vi "RGseriesSeria170309org.vi"() -> ()   [LabVIEW 2015]
uses:
  <vilib>/Instr/_visa.llb/VISA Configure Serial Port (Instr).vi
  <userlib>/caLab/Private/Get_PV.vi
panel:
  out "PS2:R_MV":dbl format="%.2f"
  out "PS1:R_MV":dbl format="%.2f"
  out "number 2":dbl
  out "number":dbl
  out "APX:Tpiezo":dbl
  in  "REMOTE/LOCAL":bool
  out "APX:Thpc":dbl
  in  "Reset Timer2":bool=TRUE caption="Auto Reset"
  in  "Time Target2 (min)":dbl=1.0 caption="Time Target (s)"
  out "Elapsed Time2 (min)":dbl caption="Elapsed Time (s)"
  out "Time has Elapsed 2":bool caption="Time has Elapsed"
  in  "Timer2":bool
  in  "Timer1":bool
  in  "Reset Timer1":bool=TRUE caption="Auto Reset"
  out "Time has Elapsed":bool
  in  "Time Target1 (min)":dbl=1.0 caption="Time Target (s)"
  out "Elapsed Time (min)":dbl caption="Elapsed Time (s)"
  in  "PS1:I_RV":dbl min=0.0 max=0.5 step=0.01
  in  "PS1:V_RV":dbl min=0.0 max=5.0 step=0.01
  out "PS1:P_MV":dbl format="%.2f"
  out "PS1:I_MV":dbl format="%.3g"
  out "PS1:V_MV":dbl format="%.3g"
  in  "PS1:OUT":bool
  out "APX:Thpc OK?":bool
  out "APX:Tpiezo OK?":bool
  out "PS2:P_MV":dbl format="%.2f"
  in  "PS2:I_RV":dbl min=0.0 max=2.3 step=0.02
  in  "PS2:OUT":bool
  in  "stop":bool
  out "PS2:I_MV":dbl format="%.3g"
  out "APX:PS2_V_MV":dbl format="%.3g"
  in  "VISA resource name":refnum<visa-resource-name>="COM12"
  in  "PS2:V_RV":dbl min=0.0 max=3.3 step=0.05
  # "COM12"
  # "Sample Heater Control"
  # "HPC Heater Control"
  # "V"
  # "V"
  # "A"
  # "A"
  # "Max 1.2A/0.4x0.1wire"
  # "W"
  # "ohm"
  # "W"
  # "ohm"
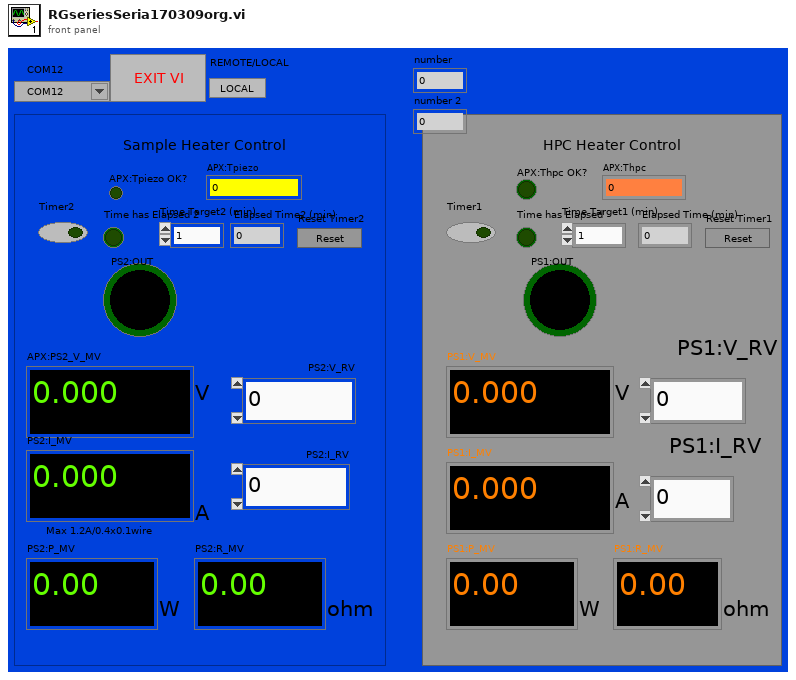
[diagram p1: front panel]
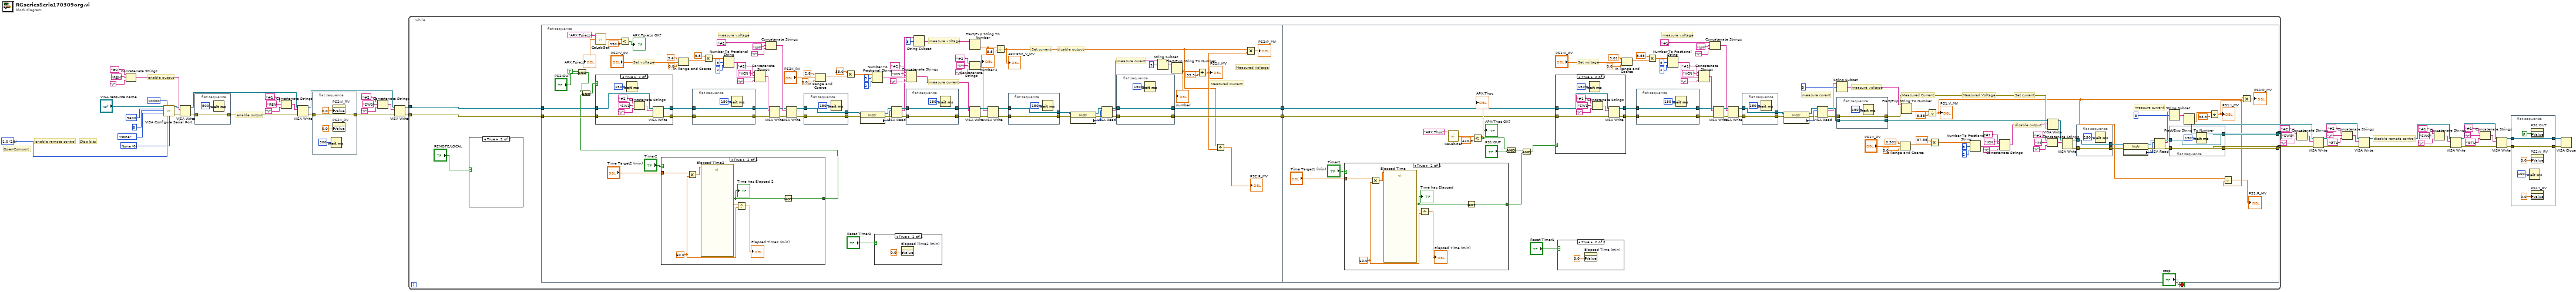
[diagram p0: block diagram]
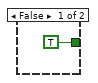
[diagram p4: hidden frame]
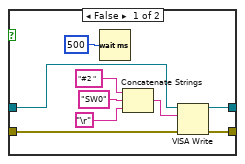
[diagram p5: hidden frame]
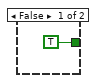
[diagram p7: hidden frame]
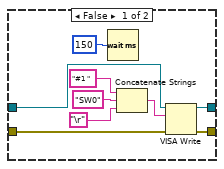
[diagram p8: hidden frame]
diagram:
  w44 = u16 0 items=["None", "XON/XOFF", "RTS/CTS", "XON/XOFF & RTS/CTS", "DTR/DSR", "XON/XOFF & DTR/DSR"] ("flow control (0:none)")
  w45 = u16 10 items=["1.0"=10, "1.5"=15, "2.0"=20] ("stop bits (10: 1 bit)")
  # "enable output"
  # "disable remote control"
  # "OpenComport"
  # "Stop bits"
  # "enable remote control"
  # "enable output"
  n1 = Concatenate Strings("#2 " ("initial string"), "REN" ("string"), "\r") -> (w43:string)
  n2 = call-poly "VISA Configure Serial Port"("VISA resource name"="VISA resource name", "timeout (10sec)"=u32 10000, "baud rate (9600)"=u32 9600, "data bits (8)"=u16 8, "parity (0:none)"=enum16{"None", "Odd", "Even", "Mark", "Space"}."None", "stop bits (10: 1 bit)"=w45, "flow control (0:none)"=w44) -> ("VISA resource name out"=w40:refnum<visa-resource-name>, "error out"=w39:errorcluster)  [unwired: 7 in]
  n3 = VISA Write(VISA resource name=w40, write buffer=w43, error in (no error)=w39) -> (VISA resource name out=w9:refnum<visa-resource-name>, error out=w2:errorcluster)  [unwired: 1 out]
  n4 = flat-sequence {
    tunnel: w2 -> [w59]
    tunnel: [w59] -> w3
    frame #0 {
      n5 = Wait (ms)(milliseconds to wait=u32 500) -> ()  [unwired: 1 out]
    }
  }
  n6 = Concatenate Strings("#1 " ("initial string"), "REN" ("string"), "\r") -> (w4:string)
  n7 = VISA Write(VISA resource name=w9, write buffer=w4, error in (no error)=w3) -> (VISA resource name out=w8:refnum<visa-resource-name>, error out=w1:errorcluster)  [unwired: 1 out]
  n8 = flat-sequence {
    tunnel: [w63] -> w26
    tunnel: w1 -> [w63]
    frame #0 {
      n9 = Wait (ms)(milliseconds to wait=u32 500) -> ()  [unwired: 1 out]
      n10 = property on="PS2:V_RV" class="DigNum (strict)"("Value"=0.0 ("VCN_REQ")) -> ()  [unwired: 2 in, 2 out]
      n11 = property on="PS2:I_RV" class="DigNum (strict)"("Value"=0.0 ("APX:RG183_I_RV")) -> ()  [unwired: 2 in, 2 out]
    }
  }
  n12 = Concatenate Strings("#2 " ("format string"), "SW0" ("initial string"), "\r" ("input 1")) -> (w42:string)
  n13 = VISA Write(VISA resource name=w8, write buffer=w42, error in (no error)=w26) -> (VISA resource name out=w28:refnum<visa-resource-name>, error out=w27:errorcluster)  [unwired: 1 out]
  n14 = while {
    tunnel: w28 -> [w70]
    tunnel: w27 -> [w71]
    tunnel: [w67] -> w25
    tunnel: [w66] -> w24
    stop <- "stop" stop-if-true
    n15 = case shown="True" "REMOTE/LOCAL" {
      frame False {
      }
      frame True {
      }
    }
    n16 = flat-sequence {
      tunnel: w71 -> [w99]
      tunnel: w70 -> [w97]
      tunnel: [w101] -> w69
      tunnel: [w100] -> w68
      tunnel: w69 -> [w243]
      tunnel: w68 -> [w240]
      tunnel: [w220] -> w67
      tunnel: [w219] -> w66
      frame #0 {
        # "measure current"
        # "measure voltage"
        # "measure voltage"
        # "measure curent"
        # "Measured Voltage"
        # "Measured Current"
        # "Set current"
        # "Set voltage"
        # "disable output"
        n17 = And(x=TRUE, y="PS2:OUT") -> (x .and. y?=w79:bool)
        n18 = call-poly <userlib>:"CaLabGet.vi"("PV Name"="APX:Tpiezo") -> ("1rst Value (number)"=w85:dbl)  [unwired: 8 in, 6 out]
        "APX:Tpiezo" <- w85
        n19 = Less?(x=w85, y=350.0) -> (x < y?=→"APX:Tpiezo OK?":bool)
        n20 = case shown="True" "Timer2" {
          tunnel: "Time Target2 (min)" -> [_ w167]
          tunnel: [TRUE w166] -> w77
          frame False {
          }
          frame True {
            w171 = 60.0 ("y")
            n21 = Multiply(x=w167, y=w171) -> (x*y=w169:dbl)
            n22 = call "Elapsed Time2"("Time Target (s)"=w169) -> ("Elapsed Time (s)"=w170:dbl, "Time has Elapsed"=w168:bool)  [unwired: 11 in, 6 out]
            "Time has Elapsed 2" <- w168
            n23 = Divide(x=w170, y=w171) -> (x/y=→"Elapsed Time2 (min)":dbl)
            n24 = Not(x=w168) -> (.not. x?=w166:bool)
          }
        }
        n25 = And(x=w79, y=w77) -> (x .and. y?=w76:bool)
        n26 = case shown="True" w76 {
          tunnel: w97 -> [w176 w185]
          tunnel: w99 -> [w175 w184]
          tunnel: [w174 w183] -> w98
          tunnel: [w173 w182] -> w96
          frame False {
            n27 = Wait (ms)(milliseconds to wait=u32 500) -> ()  [unwired: 1 out]
            n28 = Concatenate Strings("#2 " ("format string"), "SW0" ("initial string"), "\r" ("input 1")) -> (w178:string)
            n29 = VISA Write(VISA resource name=w176, write buffer=w178, error in (no error)=w175) -> (VISA resource name out=w173:refnum<visa-resource-name>, error out=w174:errorcluster)  [unwired: 1 out]
          }
          frame True {
            n30 = Wait (ms)(milliseconds to wait=u32 150) -> ()  [unwired: 1 out]
            n31 = Concatenate Strings("#2 " ("format string"), "SW1" ("initial string"), "\r" ("input 1")) -> (w187:string)
            n32 = VISA Write(VISA resource name=w185, write buffer=w187, error in (no error)=w184) -> (VISA resource name out=w182:refnum<visa-resource-name>, error out=w183:errorcluster)  [unwired: 1 out]
          }
        }
        n33 = In Range and Coerce(upper limit=3.6, x="PS2:V_RV", lower limit=0.0) -> (coerced(x)=w92:dbl)  [unwired: 1 out]
        n34 = flat-sequence {
          tunnel: w96 -> [w203]
          tunnel: w98 -> [w204]
          tunnel: [w204] -> w102
          tunnel: [w203] -> w103
          frame #0 {
            n35 = Wait (ms)(milliseconds to wait=u32 150) -> ()  [unwired: 1 out]
          }
        }
        n36 = Multiply(x=5.5, y=w92) -> (x*y=w161:dbl)
        n37 = Number To Fractional String(number=w161, width (-)=i16 5, precision (6)=i16 2) -> (F-format string=w162:string)  [unwired: 1 in]
        n38 = Concatenate Strings("#2" ("format string"), "VCN " ("initial string"), w162, "\r") -> (w107:string)
        n39 = Concatenate Strings("#2 " ("format string"), "VM" ("initial string"), "\r" ("input 1")) -> (w138:string)
        n40 = VISA Write(VISA resource name=w103, write buffer=w107, error in (no error)=w102) -> (VISA resource name out=w137:refnum<visa-resource-name>, error out=w136:errorcluster)  [unwired: 1 out]
        n41 = VISA Write(VISA resource name=w137, write buffer=w138, error in (no error)=w136) -> (VISA resource name out=w123:refnum<visa-resource-name>, error out=w121:errorcluster)  [unwired: 1 out]
        n42 = flat-sequence {
          tunnel: w123 -> [w202]
          tunnel: [w202] -> w122
          tunnel: w121 -> [w201]
          tunnel: [w201] -> w120
          frame #0 {
            n43 = Wait (ms)(milliseconds to wait=u32 150) -> ()  [unwired: 1 out]
          }
        }
        n44 = In Range and Coerce(upper limit=2.8, x="PS2:I_RV", lower limit=0.0) -> (coerced(x)=w88:dbl)  [unwired: 1 out]
        n45 = Multiply(x=33.0, y=w88) -> (x*y=w151:dbl)
        n46 = property class="Instr"(reference=w122, error in=w120) -> (reference out=w129:refnum<visa-resource-name>, error out=w128:errorcluster, "Serial Settings:Number of Bytes at Serial Port"=w127:u32)
        n47 = Number To Fractional String(number=w151, width (-)=i16 5, precision (6)=i16 2) -> (F-format string=w154:string)  [unwired: 1 in]
        n48 = case shown="True" "Reset Timer2" {
          frame False {
          }
          frame True {
            n49 = property on="Elapsed Time2 (min)" class="DigNum (strict)"("Value"=0.0 ("Elapsed Time (min)")) -> ()  [unwired: 2 in, 2 out]
          }
        }
        n50 = VISA Read(VISA resource name=w129, byte count=w127, error in (no error)=w128) -> (VISA resource name out=w115:refnum<visa-resource-name>, read buffer=w108:string, error out=w114:errorcluster)  [unwired: 1 out]
        n51 = flat-sequence {
          tunnel: w115 -> [w195]
          tunnel: w114 -> [w194]
          tunnel: [w195] -> w112
          tunnel: [w194] -> w113
          frame #0 {
            n52 = Wait (ms)(milliseconds to wait=u32 150) -> ()  [unwired: 1 out]
          }
        }
        n53 = Concatenate Strings("#2 " ("initial string"), "ICN " ("initial string"), w154, "\r") -> (w106:string)
        n54 = String Subset(string=w108, offset (0)=3) -> (substring=w105:string)  [unwired: 1 in]
        n55 = Concatenate Strings("#2 " ("format string"), "IM" ("initial string"), "\r" ("input 1")) -> (w131:string)
        n56 = Fract/Exp String To Number(string=w105) -> (number=w147:dbl)  [unwired: 3 in, 1 out]
        "number 2" <- w147
        n57 = VISA Write(VISA resource name=w112, write buffer=w106, error in (no error)=w113) -> (VISA resource name out=w133:refnum<visa-resource-name>, error out=w134:errorcluster)  [unwired: 1 out]
        n58 = VISA Write(VISA resource name=w133, write buffer=w131, error in (no error)=w134) -> (VISA resource name out=w119:refnum<visa-resource-name>, error out=w118:errorcluster)  [unwired: 1 out]
        n59 = Divide(x=w147, y=5.5 ("x")) -> (x/y=w74:dbl)
        "APX:PS2_V_MV" <- w74
        n60 = flat-sequence {
          tunnel: w119 -> [w198]
          tunnel: w118 -> [w197]
          tunnel: [w198] -> w117
          tunnel: [w197] -> w116
          frame #0 {
            n61 = Wait (ms)(milliseconds to wait=u32 150) -> ()  [unwired: 1 out]
          }
        }
        n62 = property class="Instr"(reference=w117, error in=w116) -> (reference out=w126:refnum<visa-resource-name>, error out=w125:errorcluster, "Serial Settings:Number of Bytes at Serial Port"=w124:u32)
        n63 = VISA Read(VISA resource name=w126, byte count=w124, error in (no error)=w125) -> (VISA resource name out=w111:refnum<visa-resource-name>, read buffer=w109:string, error out=w110:errorcluster)  [unwired: 1 out]
        n64 = flat-sequence {
          tunnel: w111 -> [w192]
          tunnel: w110 -> [w191]
          tunnel: [w192] -> w101
          tunnel: [w191] -> w100
          frame #0 {
            n65 = Wait (ms)(milliseconds to wait=u32 150) -> ()  [unwired: 1 out]
          }
        }
        n66 = String Subset(string=w109, offset (0)=3) -> (substring=w104:string)  [unwired: 1 in]
        n67 = Fract/Exp String To Number(string=w104) -> (number=w144:dbl)  [unwired: 3 in, 1 out]
        "number" <- w144
        n68 = Divide(x=w144, y=33.5 ("x")) -> (x/y=w75:dbl)
        "PS2:I_MV" <- w75
        n69 = Divide(x=w74, y=w75) -> (x/y=→"PS2:R_MV":dbl)
        n70 = Multiply(x=w74, y=w75) -> (x*y=→"PS2:P_MV":dbl)
      }
      frame #1 {
        # "measure curent"
        # "Measured Voltage"
        # "Measured Current"
        # "disable output"
        # "measure current"
        # "measure voltage"
        # "Set current"
        # "measure voltage"
        # "Set voltage"
        n71 = case shown="True" "Timer1" {
          tunnel: "Time Target1 (min)" -> [_ w299]
          tunnel: [TRUE w298] -> w210
          frame False {
          }
          frame True {
            w303 = 60.0 ("y")
            n72 = Multiply(x=w299, y=w303) -> (x*y=w301:dbl)
            n73 = call "Elapsed Time"("Time Target (s)"=w301) -> ("Elapsed Time (s)"=w302:dbl, "Time has Elapsed"=w300:bool)  [unwired: 11 in, 6 out]
            "Time has Elapsed" <- w300
            n74 = Divide(x=w302, y=w303) -> (x/y=→"Elapsed Time (min)":dbl)
            n75 = Not(x=w300) -> (.not. x?=w298:bool)
          }
        }
        n76 = call-poly <userlib>:"CaLabGet.vi"("PV Name"="APX:Thpc") -> ("1rst Value (number)"=w294:dbl)  [unwired: 8 in, 6 out]
        "APX:Thpc" <- w294
        n77 = Less?(x=w294, y=420.0) -> (x < y?=w242:bool)
        "APX:Thpc OK?" <- w242
        n78 = And(x=w242, y="PS1:OUT") -> (x .and. y?=w214:bool)
        n79 = And(x=w214, y=w210) -> (x .and. y?=w213:bool)
        n80 = case shown="True" w213 {
          tunnel: w243 -> [w317 w326]
          tunnel: w240 -> [w316 w325]
          tunnel: [w315 w324] -> w239
          tunnel: [w314 w323] -> w238
          frame False {
            n81 = Wait (ms)(milliseconds to wait=u32 150) -> ()  [unwired: 1 out]
            n82 = Concatenate Strings("#1 " ("format string"), "SW0" ("initial string"), "\r" ("input 1")) -> (w321:string)
            n83 = VISA Write(VISA resource name=w317, write buffer=w321, error in (no error)=w316) -> (VISA resource name out=w314:refnum<visa-resource-name>, error out=w315:errorcluster)  [unwired: 1 out]
          }
          frame True {
            n84 = Wait (ms)(milliseconds to wait=u32 150) -> ()  [unwired: 1 out]
            n85 = Concatenate Strings("#1 " ("format string"), "SW1" ("initial string"), "\r" ("input 1")) -> (w330:string)
            n86 = VISA Write(VISA resource name=w326, write buffer=w330, error in (no error)=w325) -> (VISA resource name out=w323:refnum<visa-resource-name>, error out=w324:errorcluster)  [unwired: 1 out]
          }
        }
        n87 = case shown="True" "Reset Timer1" {
          frame False {
          }
          frame True {
            n88 = property on="Elapsed Time (min)" class="DigNum (strict)"("Value"=0.0 ("Elapsed Time (min)")) -> ()  [unwired: 2 in, 2 out]
          }
        }
        n89 = In Range and Coerce(upper limit=5.01, x="PS1:V_RV", lower limit=0.0) -> (coerced(x)=w255:dbl)  [unwired: 1 out]
        n90 = flat-sequence {
          tunnel: [w333] -> w236
          tunnel: w239 -> [w333]
          tunnel: [w332] -> w237
          tunnel: w238 -> [w332]
          frame #0 {
            n91 = Wait (ms)(milliseconds to wait=u32 150) -> ()  [unwired: 1 out]
          }
        }
        n92 = Multiply(x=5.55, y=w255) -> (x*y=w246:dbl)
        n93 = Number To Fractional String(number=w246, width (-)=i16 5, precision (6)=i16 2) -> (F-format string=w245:string)  [unwired: 1 in]
        n94 = Concatenate Strings("#1" ("format string"), "VCN " ("initial string"), w245, "\r") -> (w260:string)
        n95 = Concatenate Strings("#1" ("format string"), "VM" ("initial string"), "\r" ("input 1")) -> (w259:string)
        n96 = VISA Write(VISA resource name=w237, write buffer=w260, error in (no error)=w236) -> (VISA resource name out=w261:refnum<visa-resource-name>, error out=w288:errorcluster)  [unwired: 1 out]
        n97 = VISA Write(VISA resource name=w261, write buffer=w259, error in (no error)=w288) -> (VISA resource name out=w289:refnum<visa-resource-name>, error out=w290:errorcluster)  [unwired: 1 out]
        n98 = flat-sequence {
          tunnel: w289 -> [w337]
          tunnel: [w337] -> w291
          tunnel: w290 -> [w336]
          tunnel: [w336] -> w292
          frame #0 {
            n99 = Wait (ms)(milliseconds to wait=u32 150) -> ()  [unwired: 1 out]
          }
        }
        n100 = property class="Instr"(reference=w291, error in=w292) -> (reference out=w284:refnum<visa-resource-name>, error out=w285:errorcluster, "Serial Settings:Number of Bytes at Serial Port"=w286:u32)
        n101 = VISA Read(VISA resource name=w284, byte count=w286, error in (no error)=w285) -> (VISA resource name out=w218:refnum<visa-resource-name>, read buffer=w287:string, error out=w216:errorcluster)  [unwired: 1 out]
        n102 = String Subset(string=w287, offset (0)=3) -> (substring=w276:string)  [unwired: 1 in]
        n103 = flat-sequence {
          tunnel: w218 -> [w307]
          tunnel: [w307] -> w217
          tunnel: [w305] -> w215
          tunnel: w216 -> [w305]
          frame #0 {
            n104 = Wait (ms)(milliseconds to wait=u32 150) -> ()  [unwired: 1 out]
          }
        }
        n105 = In Range and Coerce(upper limit=0.501, x="PS1:I_RV", lower limit=0.0) -> (coerced(x)=w280:dbl)  [unwired: 1 out]
        n106 = Fract/Exp String To Number(string=w276) -> (number=w270:dbl)  [unwired: 3 in, 1 out]
        n107 = Divide(x=w270, y=5.55 ("x")) -> (x/y=w208:dbl)
        "PS1:V_MV" <- w208
        n108 = Multiply(x=37.35, y=w280) -> (x*y=w266:dbl)
        n109 = Number To Fractional String(number=w266, width (-)=i16 5, precision (6)=i16 2) -> (F-format string=w263:string)  [unwired: 1 in]
        n110 = Concatenate Strings("#1 " ("initial string"), "ICN " ("initial string"), w263, "\r") -> (w281:string)
        n111 = Concatenate Strings("#1 " ("format string"), "IM" ("initial string"), "\r" ("input 1")) -> (w282:string)
        n112 = VISA Write(VISA resource name=w217, write buffer=w281, error in (no error)=w215) -> (VISA resource name out=w283:refnum<visa-resource-name>)  [unwired: 2 out]
        n113 = VISA Write(VISA resource name=w283, write buffer=w282) -> (VISA resource name out=w223:refnum<visa-resource-name>, error out=w222:errorcluster)  [unwired: 1 in, 1 out]
        n114 = flat-sequence {
          tunnel: w223 -> [w312]
          tunnel: w222 -> [w311]
          tunnel: [w312] -> w229
          tunnel: [w311] -> w228
          frame #0 {
            n115 = Wait (ms)(milliseconds to wait=u32 150) -> ()  [unwired: 1 out]
          }
        }
        n116 = property class="Instr"(reference=w229, error in=w228) -> (reference out=w232:refnum<visa-resource-name>, error out=w231:errorcluster, "Serial Settings:Number of Bytes at Serial Port"=w230:u32)
        n117 = VISA Read(VISA resource name=w232, byte count=w230, error in (no error)=w231) -> (VISA resource name out=w227:refnum<visa-resource-name>, read buffer=w225:string, error out=w226:errorcluster)  [unwired: 1 out]
        n118 = String Subset(string=w225, offset (0)=3) -> (substring=w224:string)  [unwired: 1 in]
        n119 = flat-sequence {
          tunnel: w227 -> [w309]
          tunnel: w226 -> [w308]
          tunnel: [w309] -> w220
          tunnel: [w308] -> w219
          frame #0 {
            n120 = Wait (ms)(milliseconds to wait=u32 150) -> ()  [unwired: 1 out]
          }
        }
        n121 = Fract/Exp String To Number(string=w224) -> (number=w234:dbl)  [unwired: 3 in, 1 out]
        n122 = Divide(x=w234, y=33.3 ("x")) -> (x/y=w207:dbl)
        "PS1:I_MV" <- w207
        n123 = Divide(x=w208, y=w207) -> (x/y=→"PS1:R_MV":dbl)
        n124 = Multiply(x=w208, y=w207) -> (x*y=→"PS1:P_MV":dbl)
      }
    }
  }
  n125 = Concatenate Strings("#2 " ("format string"), "SW0" ("initial string"), "\r" ("input 1")) -> (w34:string)
  n126 = VISA Write(VISA resource name=w25, write buffer=w34, error in (no error)=w24) -> (VISA resource name out=w30:refnum<visa-resource-name>, error out=w29:errorcluster)  [unwired: 1 out]
  n127 = Concatenate Strings("#2 " ("initial string"), "\r", "GTL" ("input 1")) -> (w41:string)
  n128 = VISA Write(VISA resource name=w30, write buffer=w41, error in (no error)=w29) -> (VISA resource name out=w13:refnum<visa-resource-name>, error out=w12:errorcluster)  [unwired: 1 out]
  n129 = Concatenate Strings("#1 " ("format string"), "SW0" ("initial string"), "\r" ("input 1")) -> (w19:string)
  n130 = VISA Write(VISA resource name=w13, write buffer=w19, error in (no error)=w12) -> (VISA resource name out=w15:refnum<visa-resource-name>, error out=w14:errorcluster)  [unwired: 1 out]
  n131 = Concatenate Strings("#1" ("initial string"), "\r", "GTL" ("input 1")) -> (w20:string)
  n132 = VISA Write(VISA resource name=w15, write buffer=w20, error in (no error)=w14) -> (VISA resource name out=w11:refnum<visa-resource-name>, error out=w10:errorcluster)  [unwired: 1 out]
  n133 = flat-sequence {
    tunnel: w11 -> [w342]
    tunnel: w10 -> [w341]
    tunnel: [w342] -> w36
    tunnel: [w341] -> w35
    frame #0 {
      n134 = Wait (ms)(milliseconds to wait=u32 100) -> ()  [unwired: 1 out]
      n135 = property on="PS2:OUT" class="Bool (strict)"("Value"=FALSE ("Output")) -> ()  [unwired: 2 in, 2 out]
      n136 = property on="PS2:V_RV" class="DigNum (strict)"("Value"=0.0 ("VCN_REQ")) -> ()  [unwired: 2 in, 2 out]
      n137 = property on="PS2:I_RV" class="DigNum (strict)"("Value"=0.0 ("APX:RG183_I_RV")) -> ()  [unwired: 2 in, 2 out]
    }
  }
  n138 = VISA Close(VISA resource name=w36, error in (no error)=w35) -> ()  [unwired: 1 out]
